vi "Event-View-camera-settings.vi"(8 "error in (no error)":errorcluster, 10 "Data ref. in":refnum<data-value>, 11 "UI ref. in":refnum<data-value>) -> (0 "error out":errorcluster, 2 "Data ref.":refnum<data-value>, 3 "UI ref.":refnum<data-value>)   [LabVIEW 2013, in "CameraVision.lvlib" / "CV-UI.lvclass"]
uses:
  CV-UI.lvclass
  Main/CV-Main.lvclass
  Main/Main-actions.ctl
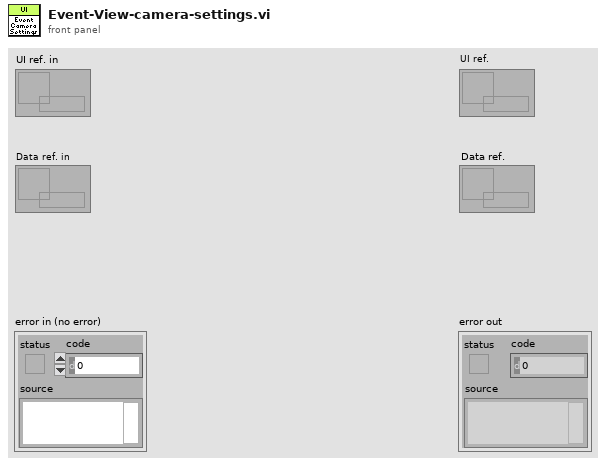
[diagram p1: front panel]
types:
  T1 = typedef "CameraVision.lvlib/CV-Main.lvclass/Main-actions.ctl" = enum16{"Idle", "Initialize", "Load defaults", "Update settings", "Check settings", "Save settings", "Save settings with dialog", "Load settings", "Load data", "Activate", "Start", "Wait for start signal", "Acquire & process", "Iterate", "Stop", "Refresh display", "Refresh status", "View camera settings", "View grabber settings", "Exit"}
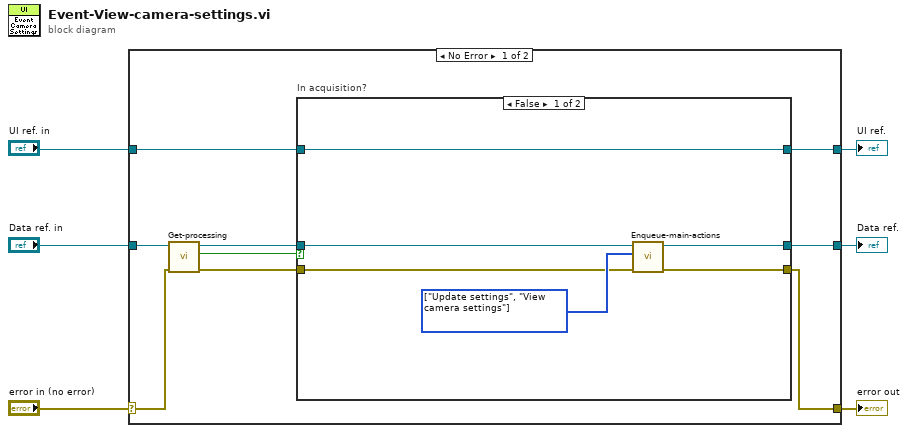
[diagram p0: block diagram]
diagram:
  n1 = case shown="No Error" "error in (no error)" {
    selector: "error in (no error)" -> [w9 w27]
    tunnel: [w7 w27] -> w5
    tunnel: [w12 w26] -> w3
    tunnel: "UI ref. in" -> [w10 w26]
    tunnel: "Data ref. in" -> [w15 w25]
    tunnel: [w11 w25] -> w1
    frame No Error {
      n2 = call "Get-processing.vi"("error in (no error)"=w9, "Data ref. in"=w15) -> ("error out"=w8:errorcluster, "Processing?"=w13:bool, "Data ref."=w14:refnum<data-value>)  [unwired: 7 in]
      n3 = case "In acquisition?" shown="False" w13 {
        tunnel: w10 -> [w21 w24]
        tunnel: w14 -> [w17 w23]
        tunnel: [w21 w24] -> w12
        tunnel: [w16 w23] -> w11
        tunnel: w8 -> [w19 w22]
        tunnel: [w18 w22] -> w7
        frame False {
          w20 = T1[] [enum."Update settings", enum."View camera settings"] items=["Idle", "Initialize", "Load defaults", "Update settings", "Check settings", "Save settings", "Save settings with dialog", "Load settings", "Load data", "Activate", "Start", "Wait for start signal", "Acquire & process", "Iterate", "Stop", "Refresh display", "Refresh status", "View camera settings", "View grabber settings", "Exit"]
          n4 = call "Enqueue-main-actions.vi"("error in (no error)"=w19, "State array"=w20, "Data ref. in"=w17) -> ("error out"=w18:errorcluster, "Data ref."=w16:refnum<data-value>)  [unwired: 6 in, 1 out]
        }
        frame True {
        }
      }
    }
    frame Error {
    }
  }
  "error out" <- w5
  "Data ref." <- w1
  "UI ref." <- w3
